vi "X_C_4352_10.vi"(0 "ek":dbl format="%#_13g", 2 "length":i32=10, 3 "q":dbl[](array[numeric])=[1.0, 1.0, 1.0, 1.0, 1.0, 1.0, 1.0, 1.0, 1.0, 1.0] format="%#_13g") -> (5 "uk":dbl format="%#_13g")   [LabVIEW 2015]
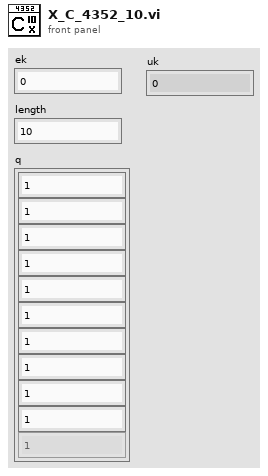
[diagram p1: front panel]
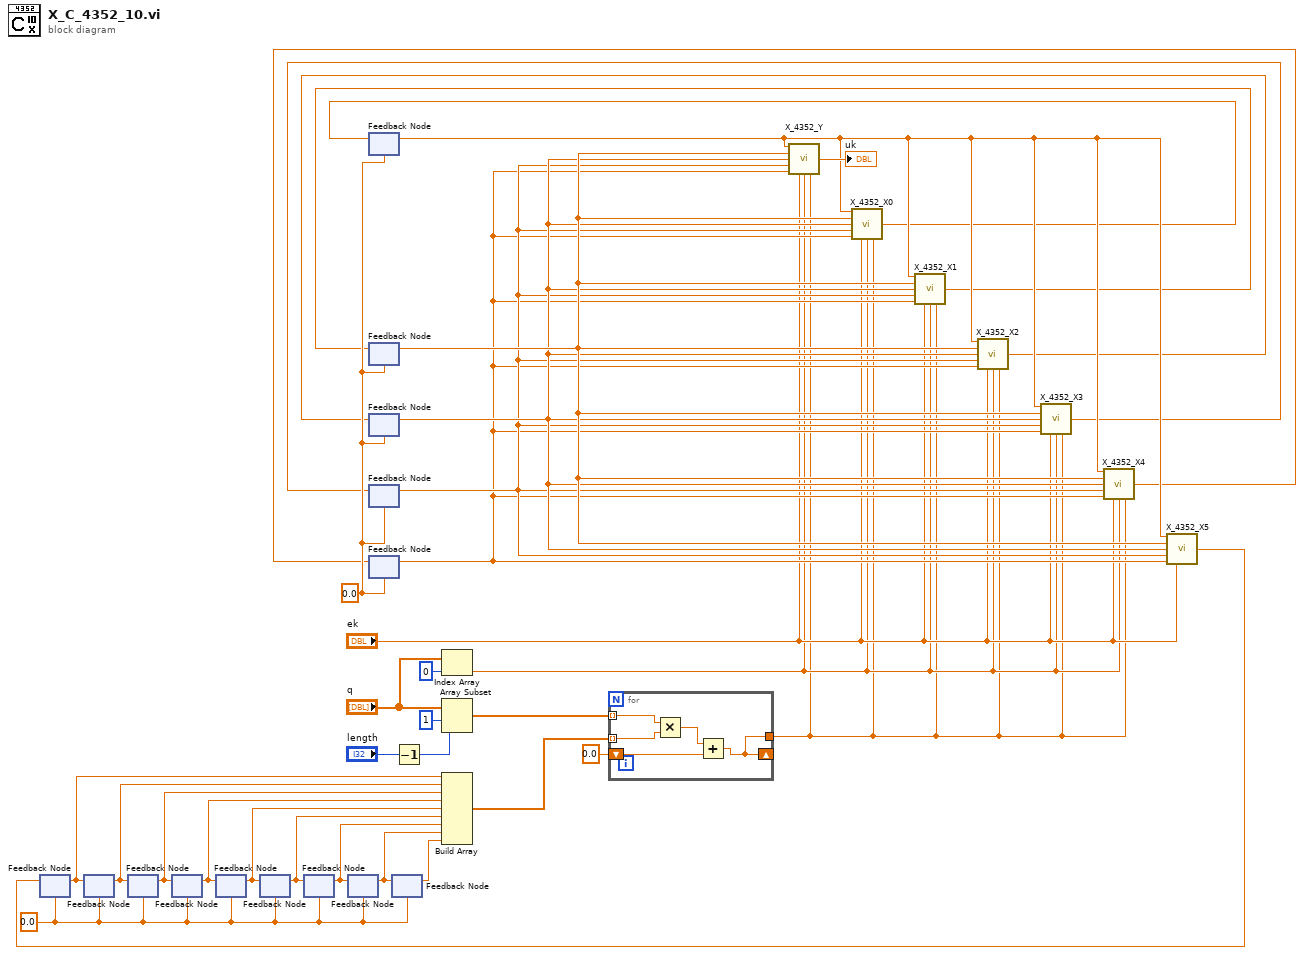
[diagram p0: block diagram]
diagram:
  w17 = 0.0
  w27 = 0.0
  n1 = feedback #1(w17) -> (w18:dbl)
  n2 = feedback #2(w17) -> (w19:dbl)
  n3 = feedback-in #2(w18) -> ()
  n4 = feedback #3(w17) -> (w20:dbl)
  n5 = feedback-in #3(w19) -> ()
  n6 = feedback #4(w17) -> (w21:dbl)
  n7 = feedback-in #4(w20) -> ()
  n8 = feedback #5(w17) -> (w22:dbl)
  n9 = feedback-in #5(w21) -> ()
  n10 = feedback #6(w17) -> (w23:dbl)
  n11 = feedback-in #6(w22) -> ()
  n12 = feedback #7(w17) -> (w24:dbl)
  n13 = feedback-in #7(w23) -> ()
  n14 = feedback #8(w17) -> (w25:dbl)
  n15 = feedback-in #8(w24) -> ()
  n16 = feedback #9(w27) -> (w14:dbl)
  n17 = feedback #10(w27) -> (w13:dbl)
  n18 = feedback #11(w27) -> (w12:dbl)
  n19 = feedback #12(w27) -> (w11:dbl)
  n20 = feedback #13(w27) -> (w10:dbl)
  n21 = feedback #14(w17) -> (w26:dbl)
  n22 = feedback-in #14(w25) -> ()
  n23 = Decrement(x="length") -> (x-1=w28:i32)
  n24 = Index Array(array="q", index=0) -> (element=w3:dbl)
  n25 = Array Subset(array="q", index=1, length=w28) -> (w29:dbl[])
  n26 = Build Array(w18, w19, w20, w21, w22, w23, w24, w25, w26) -> (w16:dbl[])
  n27 = for {
    tunnel: w16 -> [w38] mode=indexing
    tunnel: w29 -> [w39] mode=indexing
    shift-right: [w35] -> _
    shift-left: 0.0 -> [w36]
    tunnel: [w35] -> w2
    n28 = Multiply(x=w39, y=w38) -> (x*y=w37:dbl)
    n29 = Add(x=w37, y=w36) -> (x+y=w35:dbl)
  }
  n30 = call "X_4352_Y.vi"("x0"=w14, "x1"=w13, "x2"=w12, "x3"=w11, "x4"=w10, "e"="ek", "q0"=w3, "qzsum"=w2) -> ("Yout"=→"uk":dbl)  [unwired: 7 in]
  n31 = call "X_4352_X0.vi"("x0"=w14, "x1"=w13, "x2"=w12, "x3"=w11, "x4"=w10, "e"="ek", "q0"=w3, "qzsum"=w2) -> ("X0out"=w9:dbl)  [unwired: 7 in]
  n32 = feedback-in #9(w9) -> ()
  n33 = call "X_4352_X1.vi"("x0"=w14, "x1"=w13, "x2"=w12, "x3"=w11, "x4"=w10, "e"="ek", "q0"=w3, "qzsum"=w2) -> ("X1out"=w8:dbl)  [unwired: 7 in]
  n34 = feedback-in #10(w8) -> ()
  n35 = call "X_4352_X2.vi"("x0"=w14, "x1"=w13, "x2"=w12, "x3"=w11, "x4"=w10, "e"="ek", "q0"=w3, "qzsum"=w2) -> ("X2out"=w7:dbl)  [unwired: 7 in]
  n36 = feedback-in #11(w7) -> ()
  n37 = call "X_4352_X3.vi"("x0"=w14, "x1"=w13, "x2"=w12, "x3"=w11, "x4"=w10, "e"="ek", "q0"=w3, "qzsum"=w2) -> ("X3out"=w6:dbl)  [unwired: 7 in]
  n38 = feedback-in #12(w6) -> ()
  n39 = call "X_4352_X4.vi"("x0"=w14, "x1"=w13, "x2"=w12, "x3"=w11, "x4"=w10, "e"="ek", "q0"=w3, "qzsum"=w2) -> ("X4out"=w5:dbl)  [unwired: 7 in]
  n40 = feedback-in #13(w5) -> ()
  n41 = call "X_4352_X5.vi"("x0"=w14, "x1"=w13, "x2"=w12, "x3"=w11, "x4"=w10, "e"="ek") -> ("X5out"=w1:dbl)  [unwired: 9 in]
  n42 = feedback-in #1(w1) -> ()
